vi "CheckForHandicap.vi"(0 "Licence":string, 3 "error in":errorcluster, 4 "Database":string[][](array[string])) -> (10 "error out":errorcluster)   [LabVIEW 2019]
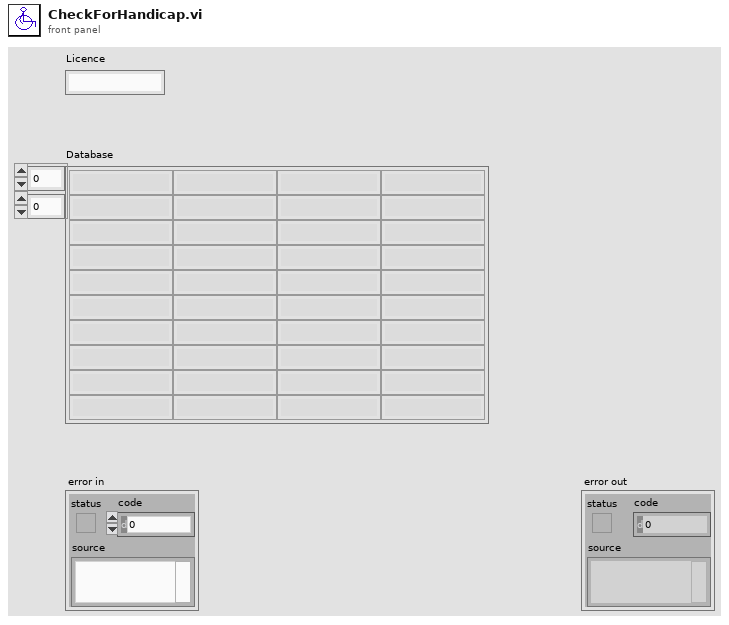
[diagram p1: front panel]
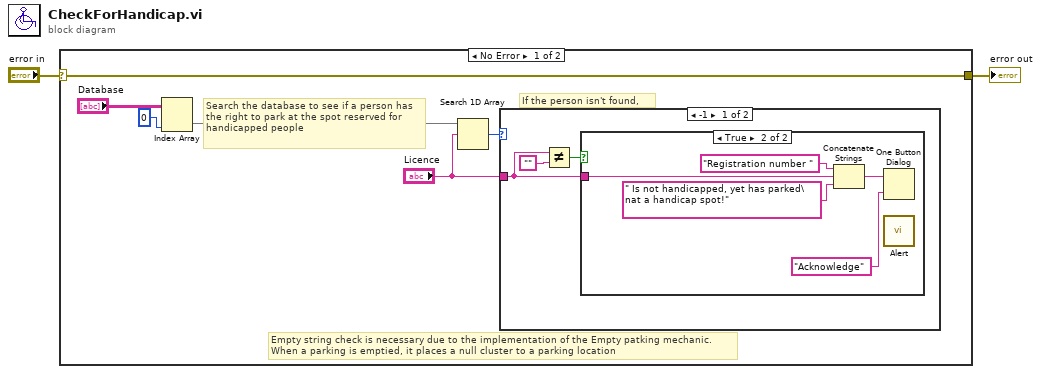
[diagram p0: block diagram]
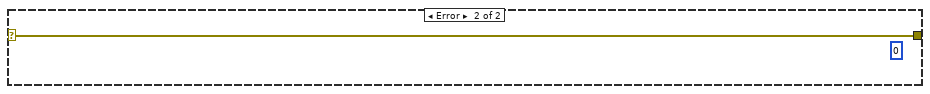
[diagram p4: hidden frame]
diagram:
  n1 = case shown="No Error" "error in" {
    selector: "error in" -> [w5 w17]
    tunnel: [w5 w17] -> w1
    frame No Error {
      # "Empty string check is necessary due to the implementation of the Empty patking mechanic.\nWhen a parking is emptied, it places a null cluster to a parking location"
      # "If the person isn't found,"
      # "Search the database to see if a person has the right to park at the spot reserved for handicapped people"
      n2 = Index Array(array="Database", index (col)=0 ("disabled index (col)")) -> (element=w8:string[])  [unwired: 1 in]
      n3 = Search 1D Array(1D array=w8, element="Licence") -> (index of element=w6:i32)  [unwired: 1 in]
      n4 = case shown="-1" w6 {
        tunnel: "Licence" -> [w10 _]
        frame -1 {
          n5 = Not Equal?(x=w10, y="") -> (x != y?=w11:bool)
          n6 = case shown="True" w11 {
            tunnel: w10 -> [_ w12]
            frame False {
            }
            frame True {
              n7 = Concatenate Strings("Registration number " ("string"), w12, " Is not handicapped, yet has parked\nat a handicap spot!" ("string")) -> (w14:string)
              n8 = One Button Dialog(message=w14, button name ("OK")="Acknowledge") -> ()  [unwired: 1 out]
              n9 = call "Alert.vi"() -> ()  [unwired: 12 in]
            }
          }
        }
        frame 1, Default {
        }
      }
    }
    frame Error {
      (unwired) 0
    }
  }
  "error out" <- w1
